vi "Find and Replace Mappings.vi"() -> ()   [LabVIEW 2025]
uses:
  <vilib>/Vehicle Communication Toolkit/TypDefs/RBS Signal.ctl
  NationalInstruments.VeriStand.SystemDefinitionAPI
  <vilib>/Vehicle Communication Toolkit/Vehicle Communication Toolkit.lvlib
panel:
  out "Array":string[](array[string])
  in  "Missing Channels with Dependencies":string[](array[string])
  out "channelPathDestinations":string[](array[string])
  out "channelPathSources":string[](array[string])
  in  "System Definition File Path":path=path "C:/Users/Nick/Desktop/VCOM Config System Definition Utility/VeriStand Example Project/Example Project/Example Project.nivssdf"
  out "error out":errorcluster
  in  "error in (no error)":errorcluster
  in  "VCOM Signal Map In":map{string, T1}(c390)
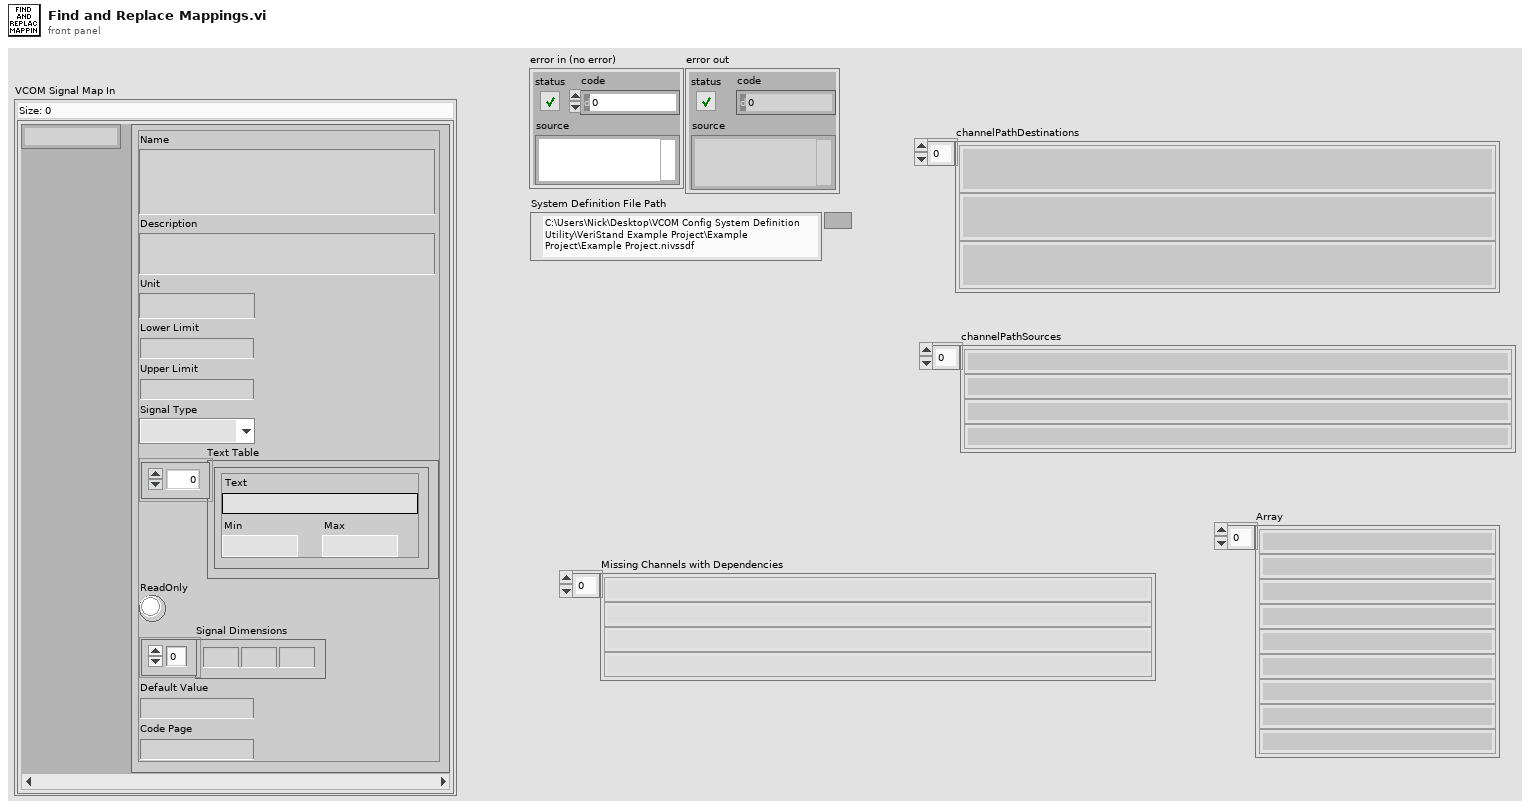
[diagram p1: front panel]
types:
  T1 = typedef "Vehicle Communication Toolkit.lvlib/RBS Signal.ctl" = cluster{"Name":string, "Description":string, "Unit":string, "Lower Limit":dbl, "Upper Limit":dbl, "Signal Type":enum32{"RE_BOOL", "RE_UINT8", "RE_INT8", "RE_UINT16", "RE_INT16", "RE_UINT32", "RE_INT32", "RE_UINT64", "RE_INT64", "RE_FLOAT32", "RE_FLOAT64", "RE_TEXT"}, "Text Table":cluster{"Text":string, "Min":dbl, "Max":dbl}[], "ReadOnly":bool, "Signal Dimensions":u32[], "Default Value":dbl, "Code Page":u32}
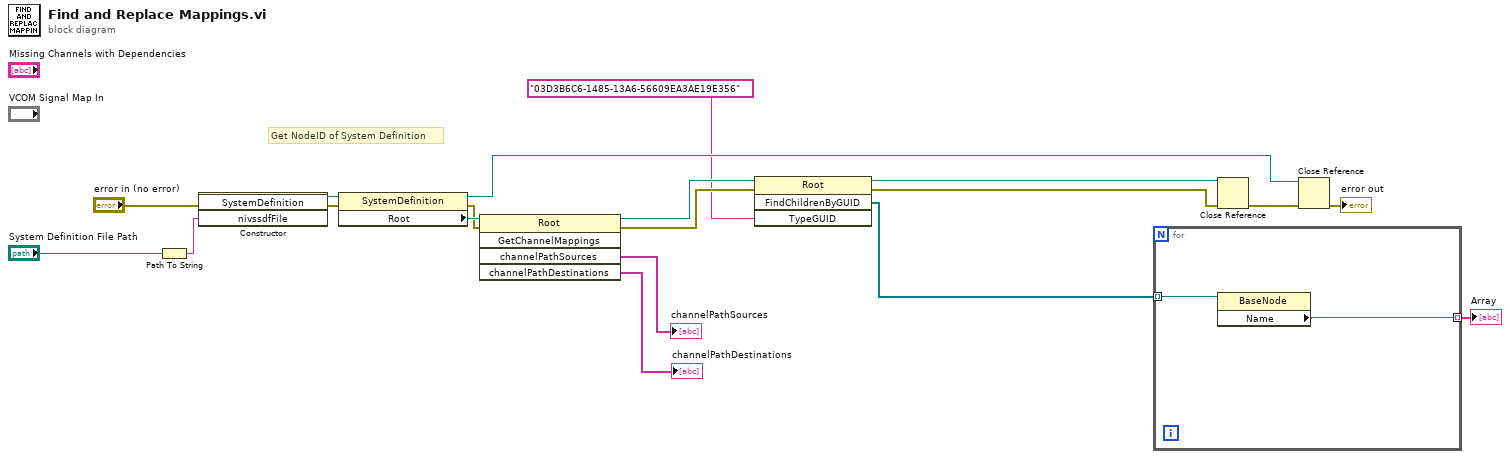
[diagram p0: block diagram]
diagram:
  # "Get NodeID of System Definition"
  n1 = Path To String(path="System Definition File Path") -> (string=w19:string)
  n2 = constructor class="SystemDefinition"(error in="error in (no error)", "nivssdfFile"=w19) -> (reference out=w17:refnum<k24>, error out=w18:errorcluster)  [unwired: 2 in, 2 out]
  n3 = property class="SystemDefinition"(reference=w17, error in=w18) -> (reference out=w14:refnum<k24>, error out=w9:errorcluster, "Root"=w12:refnum<k24>)
  n4 = invoke class="Root" method="GetChannelMappings"(reference=w12, error in=w9) -> (reference out=w6:refnum<k24>, error out=w7:errorcluster, "channelPathSources"=→"channelPathSources":string[], "channelPathDestinations"=→"channelPathDestinations":string[])  [unwired: 3 in, 1 out]
  n5 = invoke class="Root" method="FindChildrenByGUID"(reference=w6, error in=w7, "TypeGUID"="03D3B6C6-1485-13A6-56609EA3AE19E356") -> (reference out=w5:refnum<k24>, error out=w4:errorcluster, "FindChildrenByGUID"=w1:refnum<k24>[])  [unwired: 1 in, 1 out]
  n6 = for {
    tunnel: [w21] -> w3 mode=indexing
    tunnel: w1 -> [w20] mode=indexing
    n7 = property class="BaseNode"(reference=w20) -> ("Name"=w21:string)  [unwired: 1 in, 2 out]
  }
  "Array" <- w3
  n8 = Close Reference(reference=w5, error in (no error)=w4) -> (error out=w10:errorcluster)
  n9 = Close Reference(reference=w14, error in (no error)=w10) -> (error out=→"error out":errorcluster)
